vi "Prime95BCameraGrapImage.vi"(7 "error in (no error)":errorcluster, 10 "Config In":T2 {"Hardware Configuration"."Lasers Configuration"."SettingValues"."785 Power" format="%.1f"; "Hardware Configuration"."Lasers Configuration"."SettingValues"."647 Power" format="%.1f"; "Hardware Configuration"."Lasers Configuration"."SettingValues"."561 Power" format="%.1f"; "Hardware Configuration"."Lasers Configuration"."SettingValues"."532 Power" format="%.1f"; "Hardware Configuration"."Lasers Configuration"."SettingValues"."488 Power" format="%.1f"; "Hardware Configuration"."Lasers Configuration"."SettingValues"."405 Power" format="%.1f"}) -> (0 "error out":errorcluster, 2 "RawImage Out":cluster{"Time":dbl, "Image":T1}, 3 "Config Out":T2 {"Hardware Configuration"."Lasers Configuration"."SettingValues"."785 Power" format="%.1f"; "Hardware Configuration"."Lasers Configuration"."SettingValues"."647 Power" format="%.1f"; "Hardware Configuration"."Lasers Configuration"."SettingValues"."561 Power" format="%.1f"; "Hardware Configuration"."Lasers Configuration"."SettingValues"."532 Power" format="%.1f"; "Hardware Configuration"."Lasers Configuration"."SettingValues"."488 Power" format="%.1f"; "Hardware Configuration"."Lasers Configuration"."SettingValues"."405 Power" format="%.1f"})   [LabVIEW 2019]
doc: "Generates sample waveforms according to the signal type in the HW Config input."
uses:
  Settings/Settings.ctl
  Support/Hardware Configuration.ctl
  Support/Camera Configuration.ctl
  E:/DevHardSoftware/MMicroscopy/HardwareAdapter/Camera/Dependencies/PVCamNET.dll
  Dependencies/PVCamNET.dll
  <vilib>/userdefined/High Color/IMAQdx.ctl
  E:/DevHardSoftware/MMicroscopy/HardwareAdapter/Lasers/Dependencies/Oxxius_Boxx.dll
  Lasers/Dependencies/Oxxius_Boxx.dll
  Logging/Logging Configuration.ctl
  controls/UI Configuration.ctl
  <vilib>/vision/Image Controls.llb/IMAQ Image.ctl
  <vilib>/numeric/Random Number (Range) U64.vi
  <vilib>/numeric/sub_Random U32.vi
  Logging/Logging.lvlib
  Settings/Settings.lvlib
panel:
  out "Image 2":T1(plugin-control)
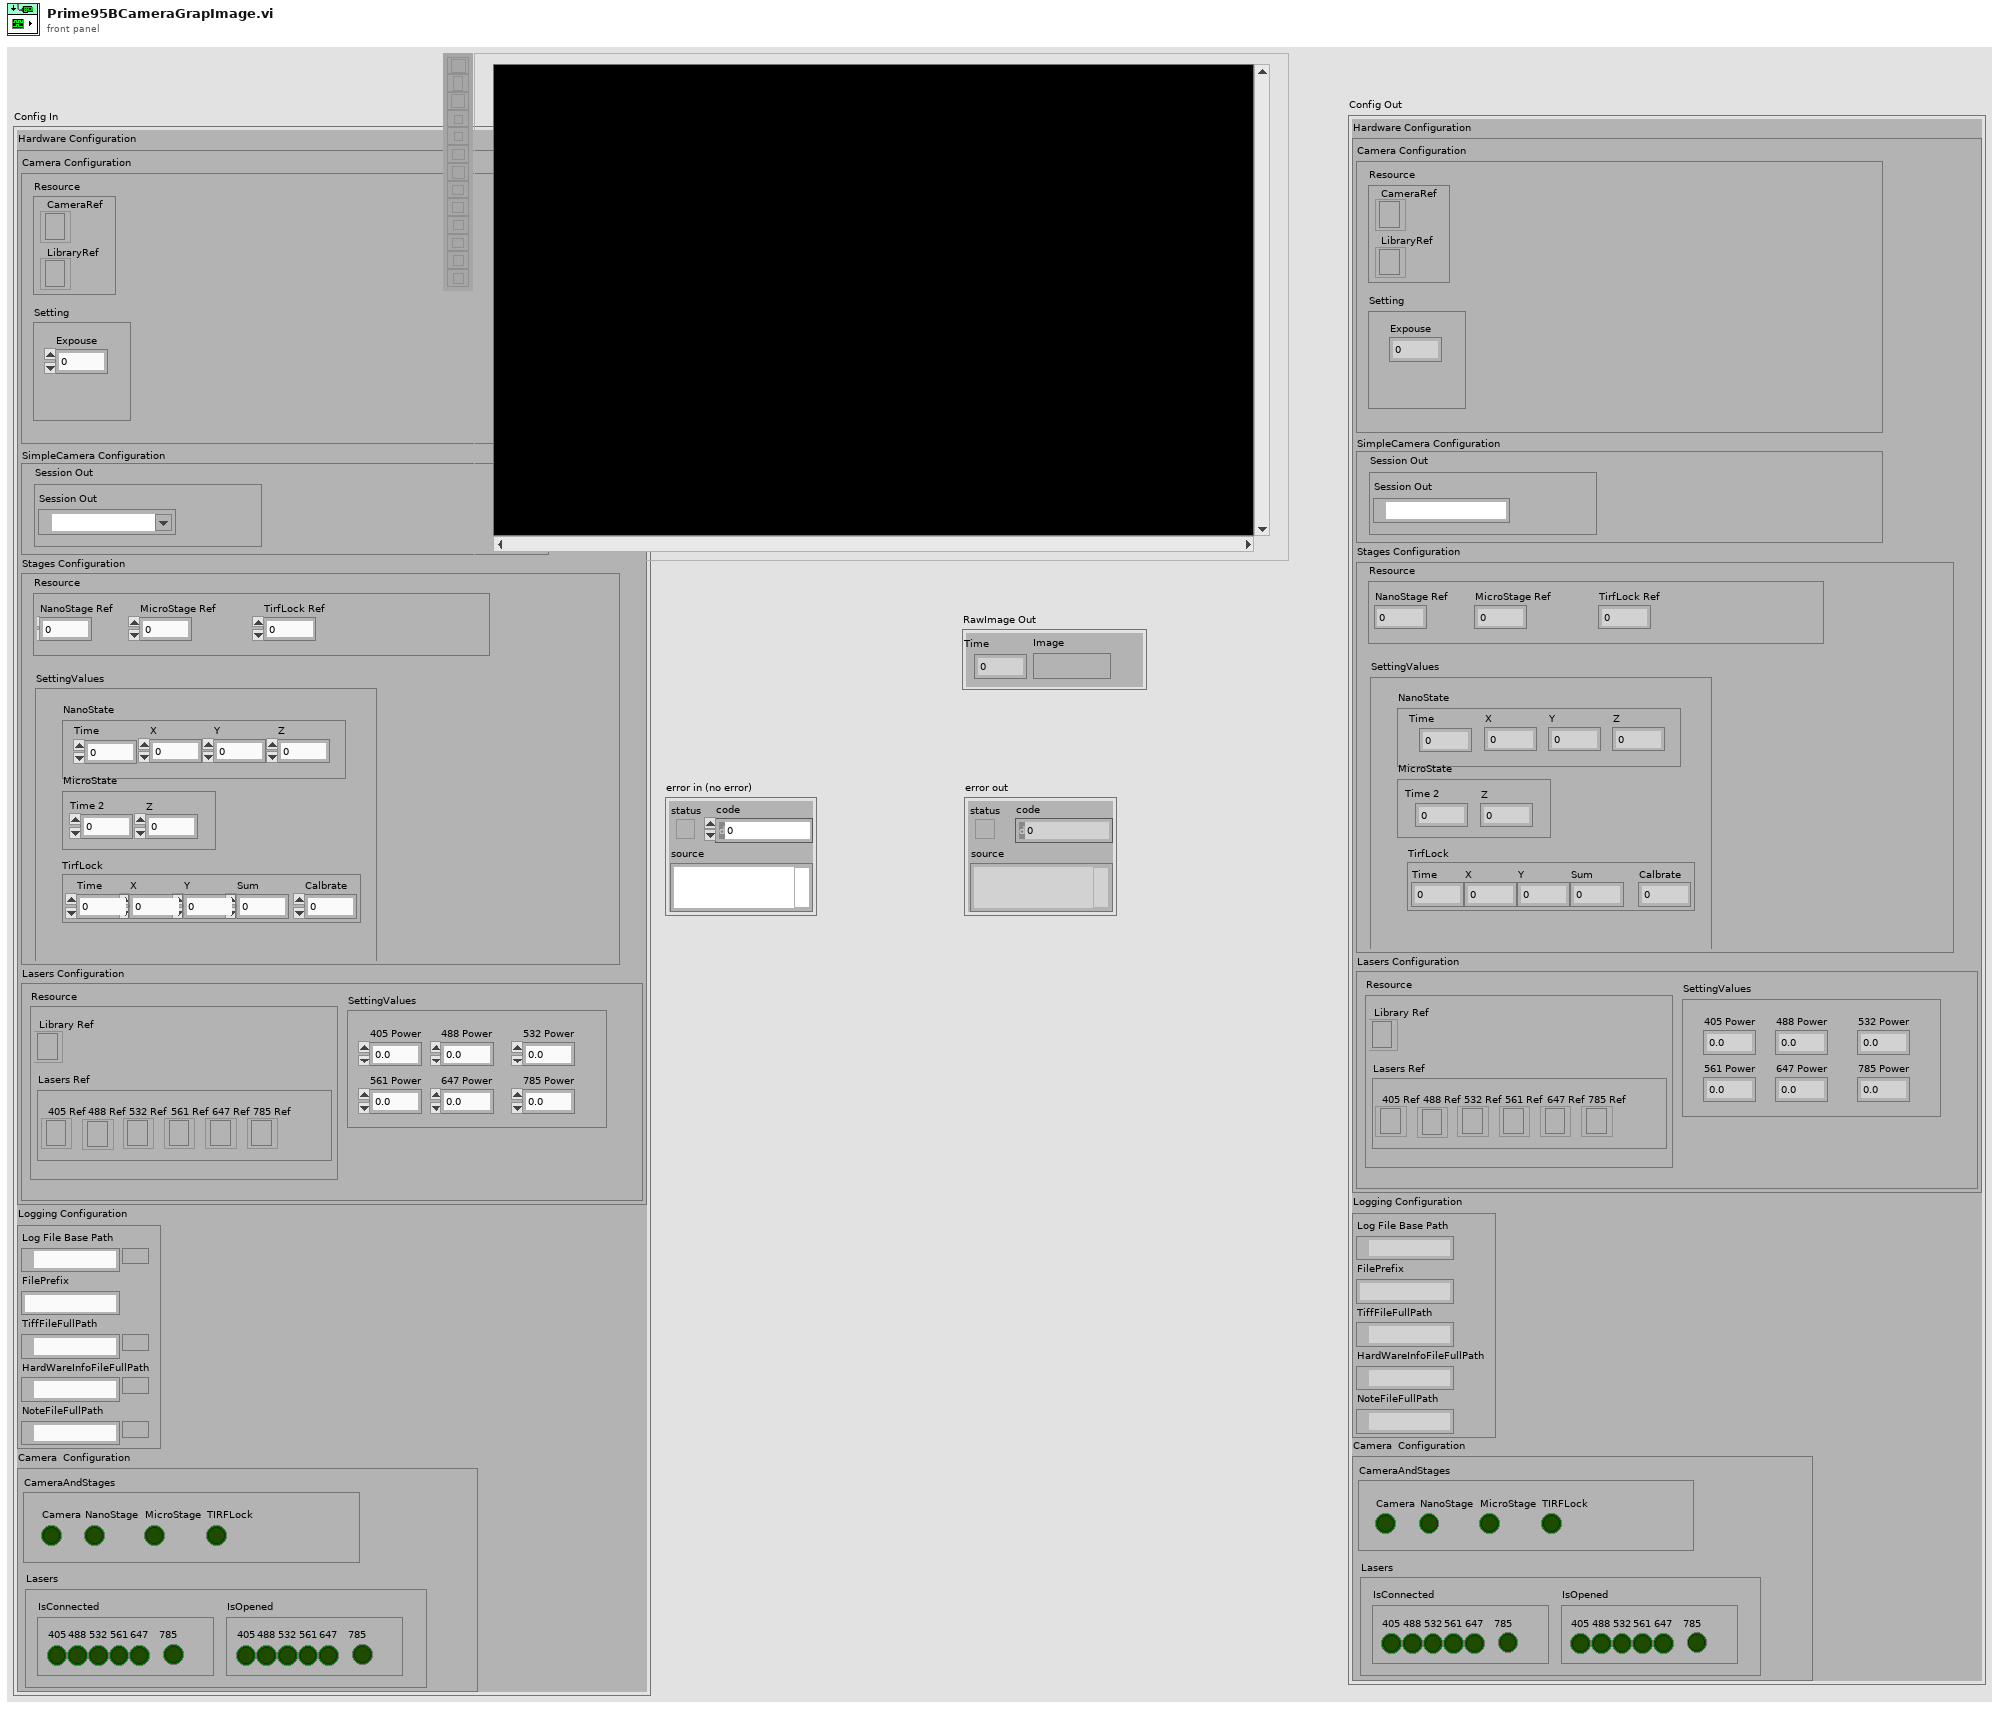
[diagram p1: front panel]
types:
  T1 = typedef "IMAQ Image.ctl" = refnum<image>
  T2 = typedef "Settings.lvlib/Settings.ctl" = cluster{"Hardware Configuration":T3, "Logging Configuration":T6, "HardWare Status":cluster{"CameraAndStages":T7, "Lasers":cluster{"IsConnected":cluster{"405":bool, "488":bool, "532":bool, "561":bool, "647":bool, "785":bool}, "IsOpened":cluster{"405":bool, "488":bool, "532":bool, "561":bool, "647":bool, "785":bool}}}}
  T3 = typedef "Hardware Configuration.ctl" = cluster{"Camera Configuration":T4, "SimpleCamera Configuration":cluster{"Resource":cluster{"Session Out":T5}}, "Stages Configuration":cluster{"Resource":cluster{"NanoStage Ref":i32, "MicroStage Ref":i32, "TirfLock Ref":i32}, "SettingValues":cluster{"NanoState":cluster{"Time":dbl, "X":dbl, "Y":dbl, "Z":dbl}, "MicroState":cluster{"Time 2":dbl, "Z":dbl}, "TirfLock":cluster{"Time":dbl, "X":dbl, "Y":dbl, "Sum":dbl, "Calbrate":dbl}}}, "Lasers Configuration":cluster{"SettingValues":cluster{"405 Power":sgl, "488 Power":sgl, "532 Power":sgl, "561 Power":sgl, "647 Power":sgl, "785 Power":sgl}, "Resource":cluster{"Library Ref":refnum<k24>, "Lasers Ref":cluster{"405 Ref":refnum<k24>, "488 Ref":refnum<k24>, "532 Ref":refnum<k24>, "561 Ref":refnum<k24>, "647 Ref":refnum<k24>, "785 Ref":refnum<k24>}}}}
  T4 = typedef "Camera Configuration.ctl" = cluster{"Resource":cluster{"CameraRef":refnum<k24>, "LibraryRef":refnum<k24>}, "Setting":cluster{"Expouse":dbl}}
  T5 = typedef "IMAQdx.ctl" = refnum<k21>
  T6 = typedef "Logging.lvlib/Logging Configuration.ctl" = cluster{"Log File Base Path":path, "FilePrefix":string, "TiffFileFullPath":path, "HardWareInfoFileFullPath":path, "NoteFileFullPath":path}
  T7 = typedef "UI Configuration.ctl" = cluster{"Camera":bool, "NanoStage":bool, "MicroStage":bool, "TIRFLock":bool}
  T8 = typedef "Image Type" = u32
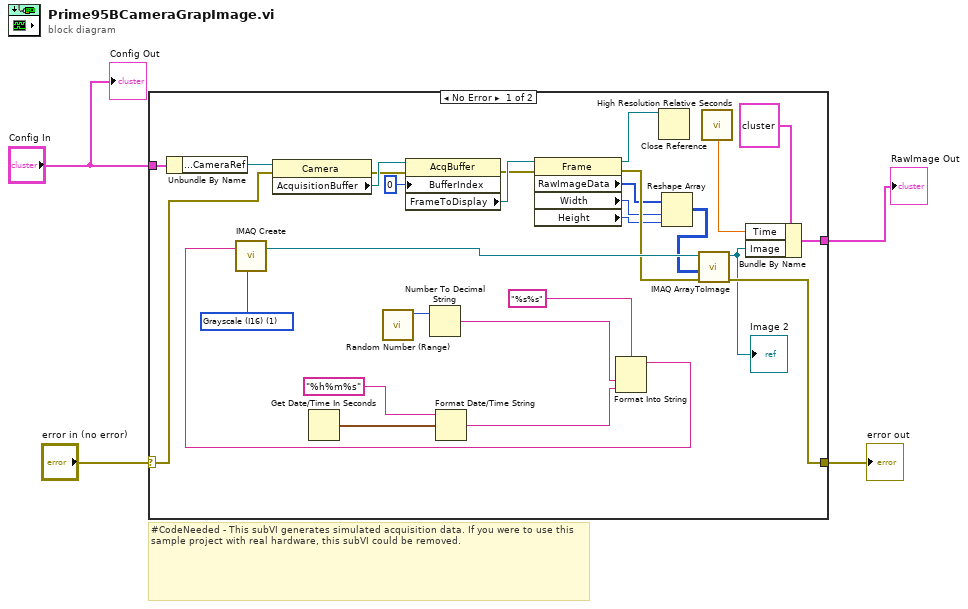
[diagram p0: block diagram]
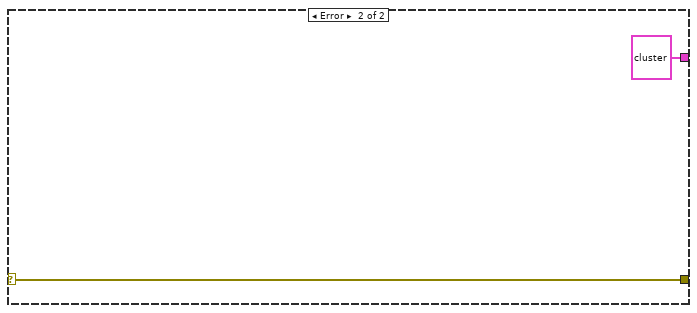
[diagram p2: hidden frame]
diagram:
  # "#CodeNeeded - This subVI generates simulated acquisition data. If you were to use this sample project with real hardware, this subVI could be removed."
  n1 = case shown="No Error" "error in (no error)" {
    selector: "error in (no error)" -> [w21 w34]
    tunnel: [w13 w34] -> w3
    tunnel: [w31 cluster{"Time":dbl, "Image":T1} {"Time"=0.0, "Image"=refnum} ("RawImage")] -> w2
    tunnel: "Config In" -> [w22 _]
    frame No Error {
      w23 = T8 1 items=["Grayscale (U8)", "Grayscale (I16)", "Grayscale (SGL)", "Complex (CSG)", "RGB (U32)", "HSL (U32)", "RGB (U64)", "Grayscale (U16)"] ("Image Type")
      n2 = Unbundle By Name(w22) -> ("Hardware Configuration.Camera Configuration.Resource.CameraRef"=w7:refnum<k24>)
      n3 = property class="Camera"(reference=w7, error in=w21) -> (error out=w19:errorcluster, "AcquisitionBuffer"=w20:refnum<k24>)  [unwired: 1 out]
      n4 = Get Date/Time In Seconds() -> (seconds since 1Jan1904=w30:timestamp)
      n5 = call-poly <vilib>:"Random Number (Range).vi"() -> ("number"=w28:u64)  [unwired: 11 in]
      n6 = property class="AcqBuffer"(reference=w20, error in=w19, "BufferIndex"=0) -> (error out=w17:errorcluster, "FrameToDisplay"=w18:refnum<k24>)  [unwired: 1 out]
      n7 = Number To Decimal String(number=w28) -> (decimal integer string=w27:string)  [unwired: 1 in]
      n8 = Format Date/Time String(time format string (%c)="%h%m%s", seconds (now)=w30) -> (date/time string=w26:string)  [unwired: 1 in]
      n9 = property class="Frame"(reference=w18, error in=w17) -> (reference out=w16:refnum<k24>, error out=w14:errorcluster, "RawImageData"=w8:i16[], "Width"=w10:u32, "Height"=w9:u32)
      n10 = Format Into String(format string="%s%s", w27, w26) -> (resulting string=w24:string)  [unwired: 2 in, 1 out]
      n11 = call "IMAQ Create"("Image Name"=w24, "Image Type"=w23) -> ("New Image"=w15:T1)  [unwired: 2 in, 2 out]
      n12 = Close Reference(reference=w16) -> ()  [unwired: 1 in, 1 out]
      n13 = Reshape Array "Reshape Array"(w8, w10, w9) -> (w5:i16[][])
      n14 = call "IMAQ ArrayToImage"("error in (no error)"=w14, "Image Pixels (I16)"=w5, "Image"=w15) -> ("error out"=w13:errorcluster, "Image Out"=w6:T1)  [unwired: 7 in]
      "Image 2" <- w6
      n15 = call <vilib>:"High Resolution Relative Seconds.vi"() -> ("relative seconds"=w12:dbl)
      n16 = Bundle By Name(cluster=cluster{"Time":dbl, "Image":T1} {"Time"=0.0, "Image"=refnum} ("RawImage"), "Time"=w12, "Image"=w6) -> (w31:cluster{"Time":dbl, "Image":T1})
    }
    frame Error {
    }
  }
  "error out" <- w3
  "RawImage Out" <- w2
  "Config Out" <- "Config In"
